vi "cube Controller.vi"(8 "error in":errorcluster) -> ()   [LabVIEW 2017]
doc: "This VI executes continuously carrying out the current operation and responding to updates or new operations. It will often contain the timing or control code that is difficult to place directly in TeleOp. This VI generally opens all sensors and motors and isolates the rest of the robot code from knowing how the operations are carried out."
uses:
  <vilib>/Rock Robotics/WPI/Framework/Completion Status.ctl
  cube Setpoints.ctl
  cube Operations.ctl
  <vilib>/Rock Robotics/WPI/MotorControl/WPI_MotorControlDeviceRef.ctl
  <vilib>/Rock Robotics/WPI/MotorControl/WPI_MotorControlType.ctl
  <vilib>/Rock Robotics/SystemInterfaces/DIO/FPGA_DIOPWMChannel.ctl
  <vilib>/Rock Robotics/WPI/PWM/WPI_PWMDeadband.ctl
  <vilib>/Rock Robotics/SystemInterfaces/DIO/FPGA_DIOChannel.ctl
  <vilib>/Rock Robotics/SystemInterfaces/AnalogTrigger/FPGA_AnalogTriggerDevRef.ctl
  <vilib>/Rock Robotics/SystemInterfaces/AnalogTrigger/FPGA_AnalogTriggerIndex.ctl
  cube Published Globals.vi
  <vilib>/Rock Robotics/SystemInterfaces/AI/FPGA_AIChannel.ctl
  Phoenix-LabVIEW/Motor Controller/Controls/CTRE_Phoenix_MotorControl_ControlMode.ctl
  Framework/Robot Global Data.vi
  <vilib>/Rock Robotics/Network Tables/NT Write Boolean.vi
panel:
  out "CubeLastCommandStatus":T1=enum."Incomplete"
  out "WaitTrigger":bool
  in  "Interactive Values":T2
  out "Current\nCmd":string
  in  "Buttons":cluster{"Execute Cmd":bool, "Abort Cmd":bool}
  out "Command Timing":cluster{"Start Time (ms)":u32, "Iterations":i32}
  out "Status":T1
  # "Tip: It may be helpful to observe inputs and sensor values.\nYou may also want to display tuning or debugging controls."
  # "Interactive Command: You may fill in the settings for a command\nand schedule it with the Execute button. You can observe and abort\nany command while fine tuning the code for the controller."
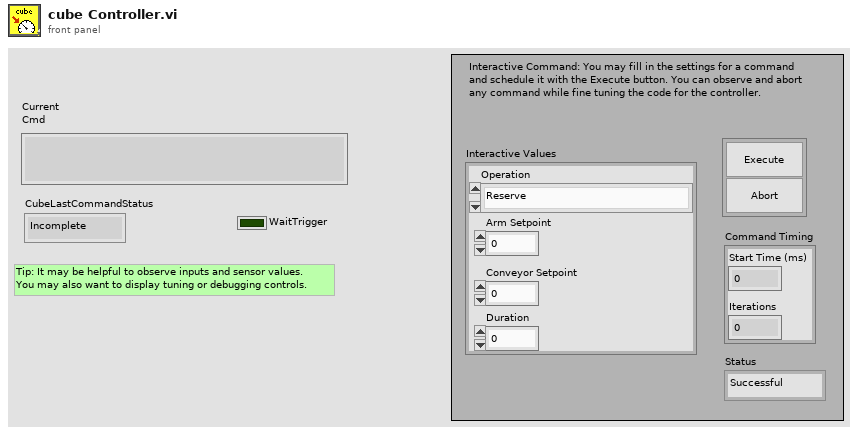
[diagram p1: front panel]
types:
  T1 = typedef "Completion Status.ctl" = enum16{"Successful", "Aborted", "Incomplete"}
  T2 = typedef "cube Setpoints.ctl" = cluster{"Operation":T3, "Arm Setpoint":dbl, "Duration":dbl, "Conveyor Setpoint":dbl}
  T3 = typedef "cube Operations.ctl" = enum16{"Reserve", "Read Current", "Immediate", "Chew", "Puke", "Swallow", "Poop", "SpitFast", "SpitSlow"}
  T4 = typedef "FPGA_AIChannel.ctl" = enum8{"AI 0", "AI 1", "AI 2", "AI 3", "AI MXP 0", "AI MXP 1", "AI MXP 2", "AI MXP 3", "Invalid"}
  T5 = typedef "FPGA_AnalogTriggerDevRef.ctl" = cluster{"DevStatus":errorcluster, "AnalogTriggerIndex":T6}
  T6 = typedef "FPGA_AnalogTriggerIndex.ctl" = enum8{"Trig 0", "Trig 1", "Trig 2", "Trig 3", "Trig 4", "Trig 5", "Trig 6", "Trig 7", "Invalid"}
  T7 = typedef "WPI_AnalogChannelDevRef.ctl" = cluster{"DevStatus":errorcluster, "Analog Channel":T4}
  T8 = typedef "WPI_MotorControlDeviceRef.ctl" = cluster{"DeviceStatus":errorcluster, "Type":T9, "PWM":cluster{"PWM Channel":T10, "DeadBand":T11}, "CAN":cluster{"Device Number":u8, "SetOutput VI Ref":variant, "GetOutput VI Ref":variant, "Enable VI Ref":variant, "Disable VI Ref":variant, "Data":variant}, "Invert":bool, "DIO PWM":cluster{"PWM \"Enable\" Channel":T10, "DIOChannel":T12, "PWM Rate":dbl}}
  T9 = typedef "WPI_MotorControlType.ctl" = enum16{"PWM", "CAN", "DIO PWM"}
  T10 = typedef "FPGA_DIOPWMChannel.ctl" = enum8{"PWM 0", "PWM 1", "PWM 2", "PWM 3", "PWM 4", "PWM 5", "PWM 6", "PWM 7", "PWM 8", "PWM 9", "PWM MXP 0", "PWM MXP 1", "PWM MXP 2", "PWM MXP 3", "PWM MXP 4", "PWM MXP 5", "PWM MXP 6", "PWM MXP 7", "PWM MXP 8", "PWM MXP 9", "Invalid"}
  T11 = typedef "WPI_PWMDeadband.ctl" = cluster{"Name":string, "maxPositivePwm":i32, "minPositivePwm":i32, "centerPwm":i32, "maxNegativePwm":i32, "minNegativePwm":i32, "angularRange":u16}
  T12 = typedef "FPGA_DIOChannel.ctl" = enum8{"DIO 0", "DIO 1", "DIO 2", "DIO 3", "DIO 4", "DIO 5", "DIO 6", "DIO 7", "DIO 8", "DIO 9", "DIO MXP 0", "DIO MXP 1", "DIO MXP 2", "DIO MXP 3", "DIO MXP 4", "DIO MXP 5", "DIO MXP 6", "DIO MXP 7", "DIO MXP 8", "DIO MXP 9", "DIO MXP 10", "DIO MXP 11", "DIO MXP 12", "DIO MXP 13", "DIO MXP 14", "DIO MXP 15", "SPI Port CS1", "SPI Port CS2", "SPI Port CS3", "SPI Port MISO", "SPI Port MOSI", "Invalid"}
  T13 = typedef "Command Status Info.ctl" = cluster{"Name":string, "Status":T1, "notifier out":T14}
  T14 = typedef "Completion Notifier.ctl" = refnum<notifier>
  T15 = cluster{"Current Command":T2, "Command Timing":cluster{"Start Time (ms)":u32, "Iterations":i32}, "Command Arguments":cluster{"Command Info":T13, "Description":string, "Default Command":T2, "queue out":refnum<queue>, "Subsystem Name":string}}
  T16 = typedef "CTRE_Phoenix_MotorControl_ControlMode.ctl" = u16
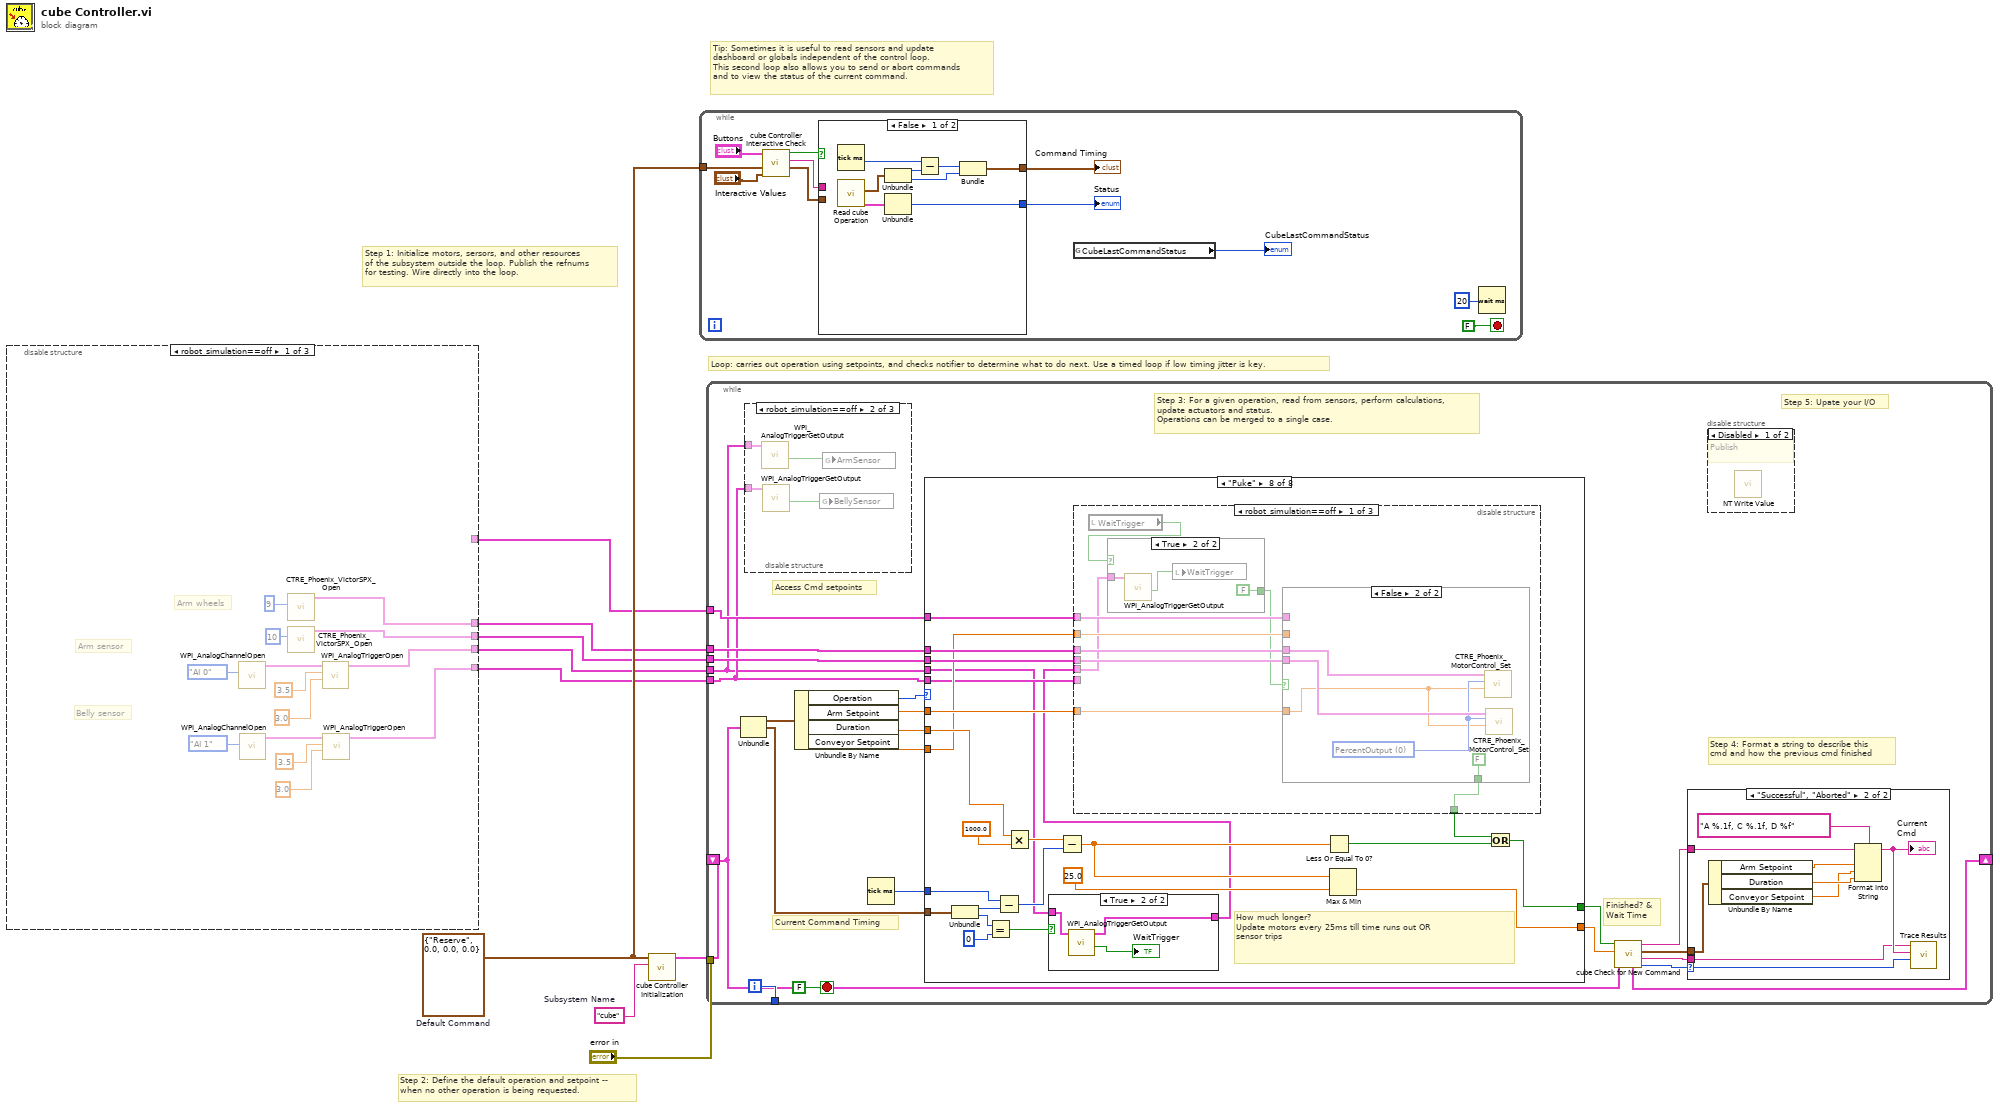
[diagram p0: block diagram]
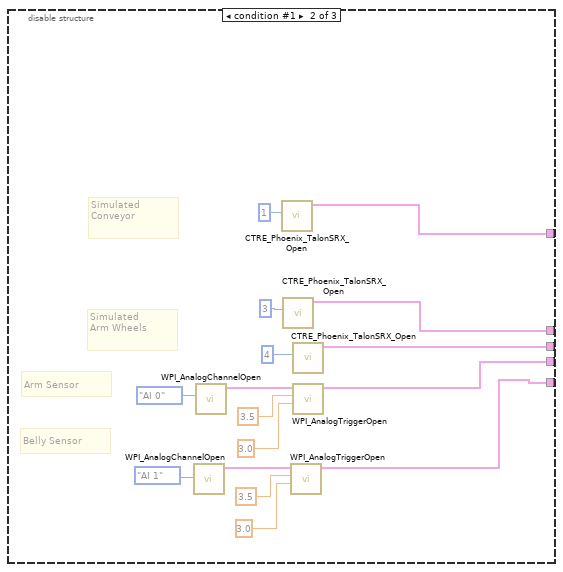
[diagram p2: hidden frame]
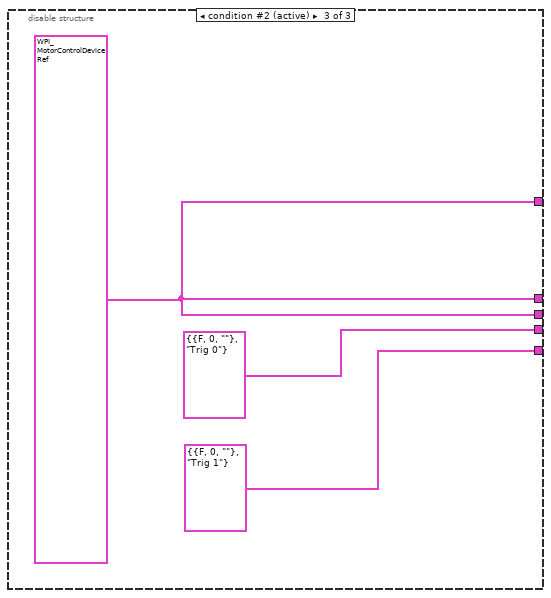
[diagram p3: hidden frame]
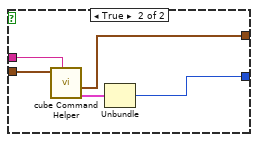
[diagram p4: hidden frame]
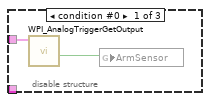
[diagram p5: hidden frame]
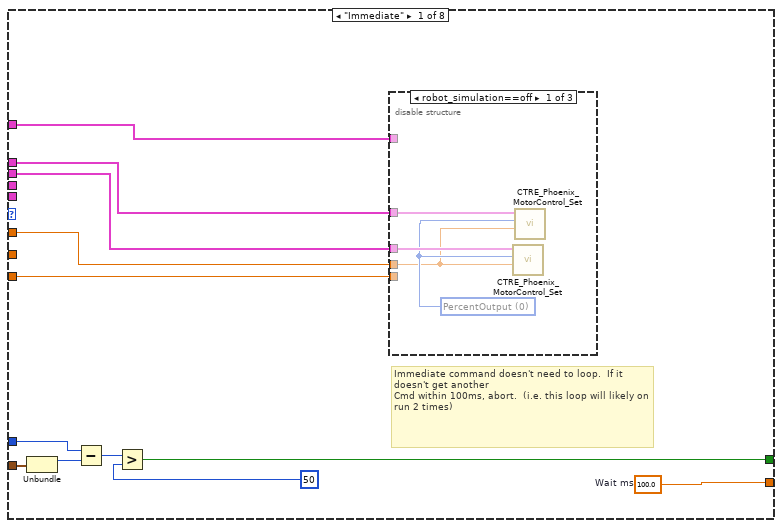
[diagram p9: hidden frame]
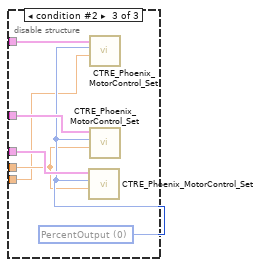
[diagram p11: hidden frame]
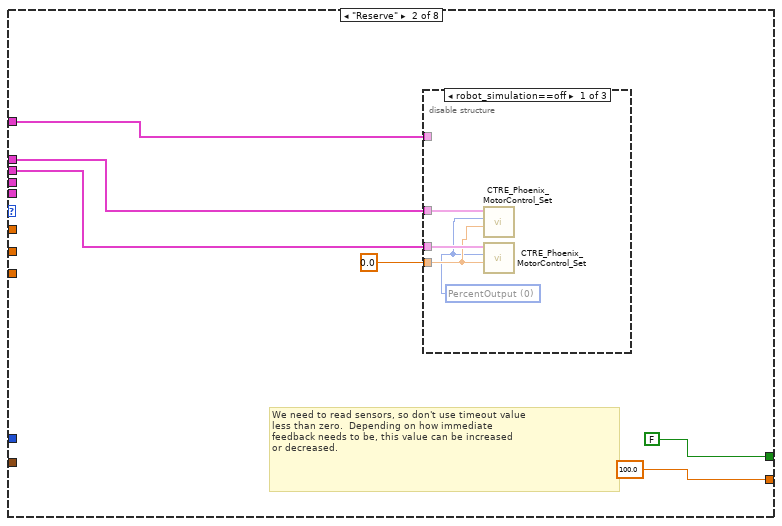
[diagram p12: hidden frame]
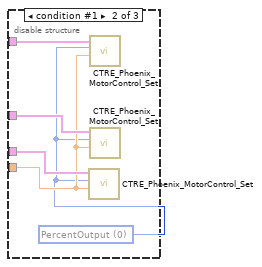
[diagram p13: hidden frame]
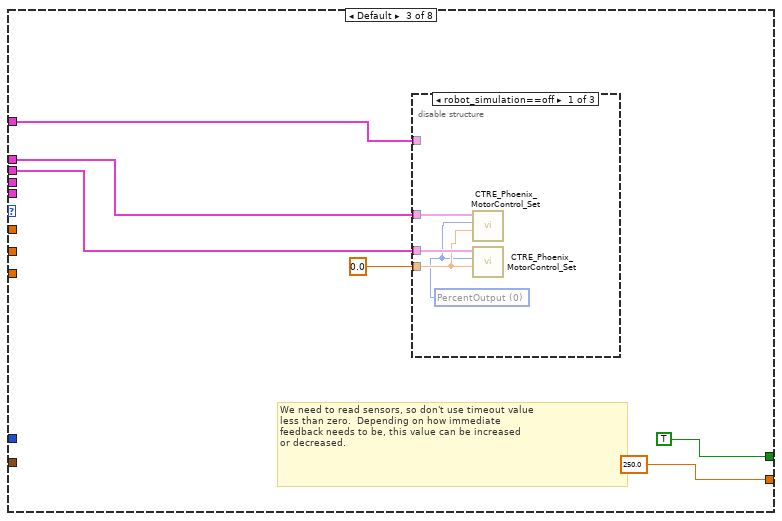
[diagram p15: hidden frame]
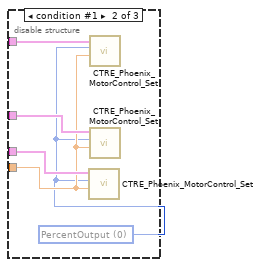
[diagram p16: hidden frame]
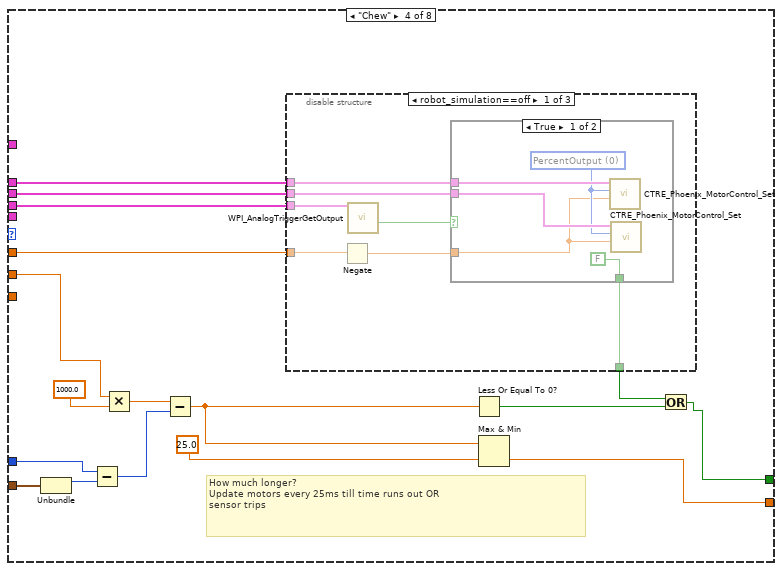
[diagram p18: hidden frame]
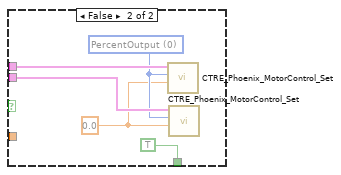
[diagram p19: hidden frame]
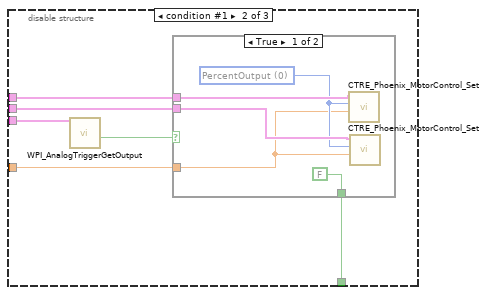
[diagram p20: hidden frame]
diagram:
  w6 = T2 {"Operation"=enum."Reserve", "Arm Setpoint"=0.0, "Duration"=0.0, "Conveyor Setpoint"=0.0}  # Default Command
  w7 = "cube"  # Subsystem Name
  # "Tip: Sometimes it is useful to read sensors and update\ndashboard or globals independent of the control loop.\nThis second loop also allows you to send or abort commands\nand to view the status of the current command."
  # "Step 2: Define the default operation and setpoint --\nwhen no other operation is being requested."
  # "Step 1: Initialize motors, sersors, and other resources\nof the subsystem outside the loop. Publish the refnums\nfor testing. Wire directly into the loop."
  # "Loop: carries out operation using setpoints, and checks notifier to determine what to do next. Use a timed loop if low timing jitter is key."
  n1 = disable-structure shown="robot_simulation==off" {
    disable-tunnel: [w21 w36 w42] -> w5
    disable-tunnel: [w20 w35 w42] -> w4
    disable-tunnel: [_ w34 w42] -> w1
    disable-tunnel: [w15 w29 T5 {"DevStatus"={"status"=FALSE, "code"=0, "source"=""}, "AnalogTriggerIndex"=enum."Trig 0"} ("AnalogTriggerDevRef")] -> w3
    disable-tunnel: [w10 w24 T5 {"DevStatus"={"status"=FALSE, "code"=0, "source"=""}, "AnalogTriggerIndex"=enum."Trig 1"} ("AnalogTriggerDevRef")] -> w2
    frame condition #0 {
      # "Belly sensor"
      # "Arm sensor"
      # "Arm wheels"
      n2 = call <vilib>:"WPI_AnalogChannelOpen.vi"("Analog Channel"=FPGA_AIChannel."AI 0") -> ("AIDeviceRef"=w18:T7)  [unwired: 9 in, 1 out]
      n3 = call <vilib>:"WPI_AnalogChannelOpen.vi"("Analog Channel"=FPGA_AIChannel."AI 1") -> ("AIDeviceRef"=w13:T7)  [unwired: 9 in, 1 out]
      n4 = call "CTRE_Phoenix_VictorSPX_Open.vi"("Device Number"=u8 9) -> ("CAN Talon SRX Ref"=w21:T8)  [unwired: 9 in, 1 out]
      n5 = call "CTRE_Phoenix_VictorSPX_Open.vi"("Device Number"=u8 10) -> ("CAN Talon SRX Ref"=w20:T8)  [unwired: 9 in, 1 out]
      n6 = call <vilib>:"WPI_AnalogTriggerOpen.vi"("LowerLimit (v)"=3.0, "UpperLimit (v)"=3.5, "AnalogTriggerSource"=w18) -> ("AnalogTriggerDevRef"=w15:T5)  [unwired: 7 in, 1 out]
      n7 = call <vilib>:"WPI_AnalogTriggerOpen.vi"("LowerLimit (v)"=3.0, "UpperLimit (v)"=3.5, "AnalogTriggerSource"=w13) -> ("AnalogTriggerDevRef"=w10:T5)  [unwired: 7 in, 1 out]
    }
    frame condition #1 {
      # "Belly Sensor"
      # "Arm Sensor"
      # "Simulated\nConveyor"
      # "Simulated\nArm Wheels"
      n8 = call <vilib>:"WPI_AnalogChannelOpen.vi"("Analog Channel"=FPGA_AIChannel."AI 1") -> ("AIDeviceRef"=w27:T7)  [unwired: 9 in, 1 out]
      n9 = call <vilib>:"WPI_AnalogChannelOpen.vi"("Analog Channel"=FPGA_AIChannel."AI 0") -> ("AIDeviceRef"=w32:T7)  [unwired: 9 in, 1 out]
      n10 = call "CTRE_Phoenix_TalonSRX_Open.vi"("Device Number"=u8 1) -> ("CAN Talon SRX Ref"=w34:T8)  [unwired: 9 in, 1 out]
      n11 = call "CTRE_Phoenix_TalonSRX_Open.vi"("Device Number"=u8 3) -> ("CAN Talon SRX Ref"=w36:T8)  [unwired: 9 in, 1 out]
      n12 = call <vilib>:"WPI_AnalogTriggerOpen.vi"("LowerLimit (v)"=3.0, "UpperLimit (v)"=3.5, "AnalogTriggerSource"=w27) -> ("AnalogTriggerDevRef"=w24:T5)  [unwired: 7 in, 1 out]
      n13 = call "CTRE_Phoenix_TalonSRX_Open.vi"("Device Number"=u8 4) -> ("CAN Talon SRX Ref"=w35:T8)  [unwired: 9 in, 1 out]
      n14 = call <vilib>:"WPI_AnalogTriggerOpen.vi"("LowerLimit (v)"=3.0, "UpperLimit (v)"=3.5, "AnalogTriggerSource"=w32) -> ("AnalogTriggerDevRef"=w29:T5)  [unwired: 7 in, 1 out]
    }
    frame condition #2 (active) {
      w42 = T8 {"DeviceStatus"={"status"=FALSE, "code"=0, "source"=""}, "Type"=enum."PWM", "PWM"={"PWM Channel"=enum."Invalid", "DeadBand"={"Name"="", "maxPositivePwm"=0, "minPositivePwm"=0, "centerPwm"=0, "maxNegativePwm"=0, "minNegativePwm"=0, "angularRange"=0}}, "CAN"={"Device Number"=0, "SetOutput VI Ref"=variant, "GetOutput VI Ref"=variant, "Enable VI Ref"=variant, "Disable VI Ref"=variant, "Data"=variant}, "Invert"=FALSE, "DIO PWM"={"PWM \"Enable\" Channel"=enum."Invalid", "DIOChannel"=enum."Invalid", "PWM Rate"=0.0}} ("CAN Talon SRX Ref")
    }
  }
  n15 = call "cube Controller Initialization.vi"("Subsystem Name"=w7, "Default Command"=w6) -> ("Current Command"=w8:T15)  [unwired: 9 in]
  n16 = while {
    tunnel: w6 -> [w50]
    stop <- FALSE stop-if-true
    n17 = call "cube Controller Interactive Check.vi"("Interactive Command in"="Interactive Values", "Default Command"=w50, "Buttons"="Buttons") -> ("Interactive Command out"=w47:T2, "Trace String"=w48:string, "Schedule"=w49:bool)  [unwired: 6 in]
    n18 = case shown="False" w49 {
      tunnel: [w61 w66] -> w46
      tunnel: w47 -> [_ w64]
      tunnel: [w57 w62] -> w45
      tunnel: w48 -> [_ w65]
      frame False {
        n19 = Tick Count (ms)() -> (millisecond timer value=w56:u32)
        n20 = call "Read cube Operation.vi"() -> ("Command Info"=w55:T13, "Command Timing"=w54:cluster{"Start Time (ms)":u32, "Iterations":i32})  [unwired: 9 in, 1 out]
        n21 = Unbundle(w54) -> ("Start Time (ms)"=w60:u32, "Iterations"=w58:i32)
        n22 = Unbundle(w55) -> ("Status"=w61:T1)  [unwired: 2 out]
        n23 = Subtract(x=w56, y=w60) -> (x-y=w59:u32)
        n24 = Bundle(w59, "Iterations"=w58) -> (w57:cluster{u32, "Iterations":i32})  [unwired: 1 in]
      }
      frame True {
        n25 = call "cube Command Helper.vi"("Description"=w65, "SubSystem Data"=w64) -> ("Command Info Out"=w63:T13, "Command Timing"=w62:cluster{"Start Time (ms)":u32, "Iterations":i32})  [unwired: 7 in, 1 out]
        n26 = Unbundle(w63) -> ("Status"=w66:T1)  [unwired: 2 out]
      }
    }
    "Status" <- w46
    "Command Timing" <- w45
    n27 = global read "cube Published Globals.vi" "CubeLastCommandStatus"() -> (→"CubeLastCommandStatus":T1)
    n28 = Wait (ms)(milliseconds to wait=u32 20) -> ()  [unwired: 1 out]
  }
  n29 = while {
    shift-right: [w84] -> _
    shift-left: w8 -> [w79]
    tunnel: [w87] -> _
    tunnel: "error in" -> [_]
    tunnel: w5 -> [w78]
    tunnel: w4 -> [w77]
    tunnel: w1 -> [w76]
    tunnel: w3 -> [w69]
    tunnel: w2 -> [w70]
    i -> [w87]
    stop <- FALSE stop-if-true
    # "Step 5: Upate your I/O"
    # "Step 4: Format a string to describe this\ncmd and how the previous cmd finished"
    # "Current Command Timing"
    # "Access Cmd setpoints"
    # "Finished? &\nWait Time"
    # "Step 3: For a given operation, read from sensors, perform calculations,\nupdate actuators and status.\nOperations can be merged to a single case."
    n30 = Unbundle(w79) -> ("Current Command"=w75:T2, "Command Timing"=w85:cluster{"Start Time (ms)":u32, "Iterations":i32})  [unwired: 1 out]
    n31 = disable-structure shown="robot_simulation==off" {
      disable-tunnel: w70 -> [_ w92 _]
      disable-tunnel: w69 -> [w89 w91 _]
      frame condition #0 {
        n32 = call <vilib>:"WPI_AnalogTriggerGetOutput.vi"("AnalogTriggerDevRef"=w89) -> ("Trigger State"=w90:bool)  [unwired: 7 in, 3 out]
        n33 = global write "Robot Global Data.vi" "ArmSensor"(w90) -> ()
      }
      frame condition #1 {
        n34 = call <vilib>:"WPI_AnalogTriggerGetOutput.vi"("AnalogTriggerDevRef"=w91) -> ("Trigger State"=w94:bool)  [unwired: 7 in, 3 out]
        n35 = call <vilib>:"WPI_AnalogTriggerGetOutput.vi"("AnalogTriggerDevRef"=w92) -> ("Trigger State"=w93:bool)  [unwired: 7 in, 3 out]
        n36 = global write "Robot Global Data.vi" "BellySensor"(w93) -> ()
        n37 = global write "Robot Global Data.vi" "ArmSensor"(w94) -> ()
      }
      frame condition #2 (active) {
      }
    }
    n38 = Unbundle By Name(w75) -> ("Operation"=w74:T3, "Arm Setpoint"=w73:dbl, "Duration"=w72:dbl, "Conveyor Setpoint"=w71:dbl)
    n39 = Tick Count (ms)() -> (millisecond timer value=w86:u32)
    n40 = case shown="\"Puke\"" w74 {
      tunnel: [w115 100.0 250.0 ("Infinite") w164 w216 w248 w278 w343] -> w67
      tunnel: [w109 FALSE ("ignore previous (F)") TRUE ("ignore previous (F)") w159 w212 w243 w274 w339] -> w68
      tunnel: w85 -> [w111 _ _ w166 w218 w250 w280 w345]
      tunnel: w86 -> [w110 _ _ w165 w217 w249 w279 w344]
      tunnel: w78 -> [w107 w128 w143 w163 w215 w247 w277 w342]
      tunnel: w77 -> [w106 w127 w142 w162 w214 w246 w276 w341]
      tunnel: w76 -> [w108 w129 w144 _ w207 _ w269 w335]
      tunnel: w73 -> [w105 _ _ w156 w209 w240 w271 w336]
      tunnel: w72 -> [_ _ _ w161 w213 w245 w275 w340]
      tunnel: w71 -> [w104 _ _ _ w206 _ w268 w334]
      tunnel: w69 -> [_ _ _ w160 _ w244 _ w329]
      tunnel: w70 -> [_ _ _ _ w208 _ w270 w333]
      frame "Immediate" {
        w115 = 100.0  # Wait ms
        # "Immediate command doesn't need to loop.  If it doesn't get another\nCmd within 100ms, abort.  (i.e. this loop will likely on run 2 times)"
        n41 = Unbundle(w111) -> ("Start Time (ms)"=w114:u32)  [unwired: 1 out]
        n42 = Subtract(x=w110, y=w114) -> (x-y=w113:u32)
        n43 = Greater?(x=w113, y=u8 50 ("Left Motor")) -> (0:w109:bool)
        n44 = disable-structure shown="robot_simulation==off" {
          disable-tunnel: w108 -> [_ _ w125]
          disable-tunnel: w107 -> [w119 _ w124]
          disable-tunnel: w106 -> [w118 _ w123]
          disable-tunnel: w105 -> [w116 _ w121]
          disable-tunnel: w104 -> [_ _ w120]
          frame condition #0 {
            w117 = T16 0 items=["PercentOutput"=0, "Position"=1, "Velocity"=2, "Current"=3, "Follower"=5, "MotionProfile"=6, "MotionMagic"=7, "MotionMagicArc"=8, "MotionProfileArc"=10, "Disabled"=15] ("Control Mode")
            n45 = call "CTRE_Phoenix_MotorControl_Set.vi"("Output"=w116, "Control Mode"=w117, "PhoenixMotorControlDevRef"=w118) -> ()  [unwired: 7 in, 2 out]
            n46 = call "CTRE_Phoenix_MotorControl_Set.vi"("Output"=w116, "Control Mode"=w117, "PhoenixMotorControlDevRef"=w119) -> ()  [unwired: 7 in, 2 out]
          }
          frame condition #1 (active) {
          }
          frame condition #2 {
            w122 = T16 0 items=["PercentOutput"=0, "Position"=1, "Velocity"=2, "Current"=3, "Follower"=5, "MotionProfile"=6, "MotionMagic"=7, "MotionMagicArc"=8, "MotionProfileArc"=10, "Disabled"=15] ("Control Mode")
            n47 = call "CTRE_Phoenix_MotorControl_Set.vi"("Output"=w121, "Control Mode"=w122, "PhoenixMotorControlDevRef"=w123) -> ()  [unwired: 7 in, 2 out]
            n48 = call "CTRE_Phoenix_MotorControl_Set.vi"("Output"=w120, "Control Mode"=w122, "PhoenixMotorControlDevRef"=w125) -> ()  [unwired: 7 in, 2 out]
            n49 = call "CTRE_Phoenix_MotorControl_Set.vi"("Output"=w121, "Control Mode"=w122, "PhoenixMotorControlDevRef"=w124) -> ()  [unwired: 7 in, 2 out]
          }
        }
      }
      frame "Reserve" {
        # "We need to read sensors, so don't use timeout value\nless than zero.  Depending on how immediate \nfeedback needs to be, this value can be increased\nor decreased."
        n50 = disable-structure shown="robot_simulation==off" {
          disable-tunnel: w129 -> [_ w140 _]
          disable-tunnel: w128 -> [w135 w139 _]
          disable-tunnel: w127 -> [w134 w138 _]
          disable-tunnel: 0.0 ("Setpoint") -> [w133 w137 _]
          frame condition #0 {
            w132 = T16 0 items=["PercentOutput"=0, "Position"=1, "Velocity"=2, "Current"=3, "Follower"=5, "MotionProfile"=6, "MotionMagic"=7, "MotionMagicArc"=8, "MotionProfileArc"=10, "Disabled"=15] ("Control Mode")
            n51 = call "CTRE_Phoenix_MotorControl_Set.vi"("Output"=w133, "Control Mode"=w132, "PhoenixMotorControlDevRef"=w135) -> ()  [unwired: 7 in, 2 out]
            n52 = call "CTRE_Phoenix_MotorControl_Set.vi"("Output"=w133, "Control Mode"=w132, "PhoenixMotorControlDevRef"=w134) -> ()  [unwired: 7 in, 2 out]
          }
          frame condition #1 {
            w136 = T16 0 items=["PercentOutput"=0, "Position"=1, "Velocity"=2, "Current"=3, "Follower"=5, "MotionProfile"=6, "MotionMagic"=7, "MotionMagicArc"=8, "MotionProfileArc"=10, "Disabled"=15] ("Control Mode")
            n53 = call "CTRE_Phoenix_MotorControl_Set.vi"("Output"=w137, "Control Mode"=w136, "PhoenixMotorControlDevRef"=w138) -> ()  [unwired: 7 in, 2 out]
            n54 = call "CTRE_Phoenix_MotorControl_Set.vi"("Output"=w137, "Control Mode"=w136, "PhoenixMotorControlDevRef"=w140) -> ()  [unwired: 7 in, 2 out]
            n55 = call "CTRE_Phoenix_MotorControl_Set.vi"("Output"=w137, "Control Mode"=w136, "PhoenixMotorControlDevRef"=w139) -> ()  [unwired: 7 in, 2 out]
          }
          frame condition #2 (active) {
          }
        }
      }
      frame Default {
        # "We need to read sensors, so don't use timeout value\nless than zero.  Depending on how immediate \nfeedback needs to be, this value can be increased\nor decreased."
        n56 = disable-structure shown="robot_simulation==off" {
          disable-tunnel: w144 -> [_ w155 _]
          disable-tunnel: w143 -> [w150 w154 _]
          disable-tunnel: w142 -> [w149 w153 _]
          disable-tunnel: 0.0 ("Setpoint") -> [w148 w152 _]
          frame condition #0 {
            w147 = T16 0 items=["PercentOutput"=0, "Position"=1, "Velocity"=2, "Current"=3, "Follower"=5, "MotionProfile"=6, "MotionMagic"=7, "MotionMagicArc"=8, "MotionProfileArc"=10, "Disabled"=15] ("Control Mode")
            n57 = call "CTRE_Phoenix_MotorControl_Set.vi"("Output"=w148, "Control Mode"=w147, "PhoenixMotorControlDevRef"=w150) -> ()  [unwired: 7 in, 2 out]
            n58 = call "CTRE_Phoenix_MotorControl_Set.vi"("Output"=w148, "Control Mode"=w147, "PhoenixMotorControlDevRef"=w149) -> ()  [unwired: 7 in, 2 out]
          }
          frame condition #1 {
            w151 = T16 0 items=["PercentOutput"=0, "Position"=1, "Velocity"=2, "Current"=3, "Follower"=5, "MotionProfile"=6, "MotionMagic"=7, "MotionMagicArc"=8, "MotionProfileArc"=10, "Disabled"=15] ("Control Mode")
            n59 = call "CTRE_Phoenix_MotorControl_Set.vi"("Output"=w152, "Control Mode"=w151, "PhoenixMotorControlDevRef"=w153) -> ()  [unwired: 7 in, 2 out]
            n60 = call "CTRE_Phoenix_MotorControl_Set.vi"("Output"=w152, "Control Mode"=w151, "PhoenixMotorControlDevRef"=w155) -> ()  [unwired: 7 in, 2 out]
            n61 = call "CTRE_Phoenix_MotorControl_Set.vi"("Output"=w152, "Control Mode"=w151, "PhoenixMotorControlDevRef"=w154) -> ()  [unwired: 7 in, 2 out]
          }
          frame condition #2 (active) {
          }
        }
      }
      frame "Chew" {
        # "How much longer?\nUpdate motors every 25ms till time runs out OR\nsensor trips"
        n62 = Unbundle(w166) -> ("Start Time (ms)"=w169:u32)  [unwired: 1 out]
        n63 = Subtract(x=w165, y=w169) -> (x-y=w172:u32)
        n64 = Multiply(x=w161, y=1000.0) -> (x*y=w171:dbl)
        n65 = Subtract(x=w171, y=w172) -> (x-y=w168:dbl)
        n66 = disable-structure shown="robot_simulation==off" {
          disable-tunnel: w163 -> [w179 w195 _]
          disable-tunnel: w162 -> [w178 w194 _]
          disable-tunnel: w156 -> [w173 w193 _]
          disable-tunnel: w160 -> [w177 w192 _]
          disable-tunnel: [w175 w190 _] -> w157
          frame condition #0 {
            n67 = Negate(x=w173) -> (-x=w174:dbl)
            n68 = call <vilib>:"WPI_AnalogTriggerGetOutput.vi"("AnalogTriggerDevRef"=w177) -> ("Trigger State"=w176:bool)  [unwired: 7 in, 3 out]
            n69 = case shown="True" w176 {
              tunnel: w179 -> [w184 w189]
              tunnel: w178 -> [w183 w188]
              tunnel: w174 -> [w180 _]
              tunnel: [FALSE TRUE] -> w175
              frame True {
                w182 = T16 0 items=["PercentOutput"=0, "Position"=1, "Velocity"=2, "Current"=3, "Follower"=5, "MotionProfile"=6, "MotionMagic"=7, "MotionMagicArc"=8, "MotionProfileArc"=10, "Disabled"=15] ("Control Mode")
                n70 = call "CTRE_Phoenix_MotorControl_Set.vi"("Output"=w180, "Control Mode"=w182, "PhoenixMotorControlDevRef"=w184) -> ()  [unwired: 7 in, 2 out]
                n71 = call "CTRE_Phoenix_MotorControl_Set.vi"("Output"=w180, "Control Mode"=w182, "PhoenixMotorControlDevRef"=w183) -> ()  [unwired: 7 in, 2 out]
              }
              frame False {
                w186 = 0.0 ("Output")
                w187 = T16 0 items=["PercentOutput"=0, "Position"=1, "Velocity"=2, "Current"=3, "Follower"=5, "MotionProfile"=6, "MotionMagic"=7, "MotionMagicArc"=8, "MotionProfileArc"=10, "Disabled"=15] ("Control Mode")
                n72 = call "CTRE_Phoenix_MotorControl_Set.vi"("Output"=w186, "Control Mode"=w187, "PhoenixMotorControlDevRef"=w189) -> ()  [unwired: 7 in, 2 out]
                n73 = call "CTRE_Phoenix_MotorControl_Set.vi"("Output"=w186, "Control Mode"=w187, "PhoenixMotorControlDevRef"=w188) -> ()  [unwired: 7 in, 2 out]
              }
            }
          }
          frame condition #1 {
            n74 = call <vilib>:"WPI_AnalogTriggerGetOutput.vi"("AnalogTriggerDevRef"=w192) -> ("Trigger State"=w191:bool)  [unwired: 7 in, 3 out]
            n75 = case shown="True" w191 {
              tunnel: w195 -> [w199 w205]
              tunnel: w194 -> [w198 w204]
              tunnel: w193 -> [w196 _]
              tunnel: [FALSE TRUE] -> w190
              frame True {
                w197 = T16 0 items=["PercentOutput"=0, "Position"=1, "Velocity"=2, "Current"=3, "Follower"=5, "MotionProfile"=6, "MotionMagic"=7, "MotionMagicArc"=8, "MotionProfileArc"=10, "Disabled"=15] ("Control Mode")
                n76 = call "CTRE_Phoenix_MotorControl_Set.vi"("Output"=w196, "Control Mode"=w197, "PhoenixMotorControlDevRef"=w199) -> ()  [unwired: 7 in, 2 out]
                n77 = call "CTRE_Phoenix_MotorControl_Set.vi"("Output"=w196, "Control Mode"=w197, "PhoenixMotorControlDevRef"=w198) -> ()  [unwired: 7 in, 2 out]
              }
              frame False {
                w203 = T16 0 items=["PercentOutput"=0, "Position"=1, "Velocity"=2, "Current"=3, "Follower"=5, "MotionProfile"=6, "MotionMagic"=7, "MotionMagicArc"=8, "MotionProfileArc"=10, "Disabled"=15] ("Control Mode")
                w202 = 0.0 ("Output")
                n78 = call "CTRE_Phoenix_MotorControl_Set.vi"("Output"=w202, "Control Mode"=w203, "PhoenixMotorControlDevRef"=w205) -> ()  [unwired: 7 in, 2 out]
                n79 = call "CTRE_Phoenix_MotorControl_Set.vi"("Output"=w202, "Control Mode"=w203, "PhoenixMotorControlDevRef"=w204) -> ()  [unwired: 7 in, 2 out]
              }
            }
          }
          frame condition #2 (active) {
          }
        }
        n80 = Less Or Equal To 0?(x=w168) -> (x <= 0?=w158:bool)
        n81 = Max & Min(x=w168, y=25.0) -> (min(x,y)=w164:dbl)  [unwired: 1 out]
        n82 = Or(x=w157, y=w158) -> (x .or. y?=w159:bool)
      }
      frame "Poop" {
        # "How much longer?\nUpdate motors every 25ms till time runs out OR\nsensor trips"
        n83 = Unbundle(w218) -> ("Start Time (ms)"=w221:u32)  [unwired: 1 out]
        n84 = Subtract(x=w217, y=w221) -> (x-y=w224:u32)
        n85 = Multiply(x=w213, y=1000.0) -> (x*y=w223:dbl)
        n86 = Subtract(x=w223, y=w224) -> (x-y=w220:dbl)
        n87 = disable-structure shown="robot_simulation==off" {
          disable-tunnel: w215 -> [w230 w239 _]
          disable-tunnel: w214 -> [w229 w238 _]
          disable-tunnel: w209 -> [w227 w234 _]
          disable-tunnel: w208 -> [_ _ _]
          disable-tunnel: [FALSE FALSE _] -> w210
          disable-tunnel: w207 -> [_ w236 _]
          disable-tunnel: w206 -> [_ w233 _]
          frame condition #0 {
            w226 = T16 0 items=["PercentOutput"=0, "Position"=1, "Velocity"=2, "Current"=3, "Follower"=5, "MotionProfile"=6, "MotionMagic"=7, "MotionMagicArc"=8, "MotionProfileArc"=10, "Disabled"=15] ("Control Mode")
            n88 = Negate(x=w227) -> (-x=w225:dbl)
            n89 = call "CTRE_Phoenix_MotorControl_Set.vi"("Output"=w225, "Control Mode"=w226, "PhoenixMotorControlDevRef"=w230) -> ()  [unwired: 7 in, 2 out]
            n90 = call "CTRE_Phoenix_MotorControl_Set.vi"("Output"=w225, "Control Mode"=w226, "PhoenixMotorControlDevRef"=w229) -> ()  [unwired: 7 in, 2 out]
          }
          frame condition #1 {
            w235 = T16 0 items=["PercentOutput"=0, "Position"=1, "Velocity"=2, "Current"=3, "Follower"=5, "MotionProfile"=6, "MotionMagic"=7, "MotionMagicArc"=8, "MotionProfileArc"=10, "Disabled"=15] ("Control Mode")
            n91 = Negate(x=w234) -> (-x=w231:dbl)
            n92 = Negate(x=w233) -> (-x=w232:dbl)
            n93 = call "CTRE_Phoenix_MotorControl_Set.vi"("Output"=w231, "Control Mode"=w235, "PhoenixMotorControlDevRef"=w239) -> ()  [unwired: 7 in, 2 out]
            n94 = call "CTRE_Phoenix_MotorControl_Set.vi"("Output"=w231, "Control Mode"=w235, "PhoenixMotorControlDevRef"=w238) -> ()  [unwired: 7 in, 2 out]
            n95 = call "CTRE_Phoenix_MotorControl_Set.vi"("Output"=w232, "Control Mode"=w235, "PhoenixMotorControlDevRef"=w236) -> ()  [unwired: 7 in, 2 out]
          }
          frame condition #2 (active) {
          }
        }
        n96 = Less Or Equal To 0?(x=w220) -> (x <= 0?=w211:bool)
        n97 = Max & Min(x=w220, y=25.0) -> (min(x,y)=w216:dbl)  [unwired: 1 out]
        n98 = Or(x=w210, y=w211) -> (x .or. y?=w212:bool)
      }
      frame "SpitFast" {
        # "How much longer?\nUpdate motors every 25ms till time runs out OR\nsensor trips"
        n99 = Unbundle(w250) -> ("Start Time (ms)"=w253:u32)  [unwired: 1 out]
        n100 = Subtract(x=w249, y=w253) -> (x-y=w256:u32)
        n101 = Multiply(x=w245, y=1000.0) -> (x*y=w255:dbl)
        n102 = Subtract(x=w255, y=w256) -> (x-y=w252:dbl)
        n103 = disable-structure shown="robot_simulation==off" {
          disable-tunnel: w247 -> [w261 w267 _]
          disable-tunnel: w246 -> [w260 w266 _]
          disable-tunnel: w240 -> [w257 w264 _]
          disable-tunnel: w244 -> [_ _ _]
          disable-tunnel: [FALSE FALSE _] -> w241
          frame condition #0 {
            w258 = T16 0 items=["PercentOutput"=0, "Position"=1, "Velocity"=2, "Current"=3, "Follower"=5, "MotionProfile"=6, "MotionMagic"=7, "MotionMagicArc"=8, "MotionProfileArc"=10, "Disabled"=15] ("Control Mode")
            n104 = call "CTRE_Phoenix_MotorControl_Set.vi"("Output"=w257, "Control Mode"=w258, "PhoenixMotorControlDevRef"=w261) -> ()  [unwired: 7 in, 2 out]
            n105 = call "CTRE_Phoenix_MotorControl_Set.vi"("Output"=w257, "Control Mode"=w258, "PhoenixMotorControlDevRef"=w260) -> ()  [unwired: 7 in, 2 out]
          }
          frame condition #1 {
            w263 = T16 0 items=["PercentOutput"=0, "Position"=1, "Velocity"=2, "Current"=3, "Follower"=5, "MotionProfile"=6, "MotionMagic"=7, "MotionMagicArc"=8, "MotionProfileArc"=10, "Disabled"=15] ("Control Mode")
            n106 = Negate(x=w264) -> (-x=w262:dbl)
            n107 = call "CTRE_Phoenix_MotorControl_Set.vi"("Output"=w262, "Control Mode"=w263, "PhoenixMotorControlDevRef"=w267) -> ()  [unwired: 7 in, 2 out]
            n108 = call "CTRE_Phoenix_MotorControl_Set.vi"("Output"=w262, "Control Mode"=w263, "PhoenixMotorControlDevRef"=w266) -> ()  [unwired: 7 in, 2 out]
          }
          frame condition #2 (active) {
          }
        }
        n109 = Less Or Equal To 0?(x=w252) -> (x <= 0?=w242:bool)
        n110 = Max & Min(x=w252, y=25.0) -> (min(x,y)=w248:dbl)  [unwired: 1 out]
        n111 = Or(x=w241, y=w242) -> (x .or. y?=w243:bool)
      }
      frame "Swallow" {
        # "How much longer?\nUpdate motors every 25ms till time runs out OR\nsensor trips"
        n112 = Unbundle(w280) -> ("Start Time (ms)"=w283:u32)  [unwired: 1 out]
        n113 = Subtract(x=w279, y=w283) -> (x-y=w286:u32)
        n114 = Multiply(x=w275, y=1000.0) -> (x*y=w285:dbl)
        n115 = Subtract(x=w285, y=w286) -> (x-y=w282:dbl)
        n116 = disable-structure shown="robot_simulation==off" {
          disable-tunnel: w277 -> [w293 w314 _]
          disable-tunnel: w276 -> [w292 w313 _]
          disable-tunnel: w271 -> [w288 w312 _]
          disable-tunnel: w270 -> [w295 w311 _]
          disable-tunnel: [w291 w309 _] -> w272
          disable-tunnel: w269 -> [w294 w308 _]
          disable-tunnel: w268 -> [w289 w307 _]
          frame condition #0 {
            n117 = Negate(x=w288) -> (-x=w287:dbl)
            n118 = call <vilib>:"WPI_AnalogTriggerGetOutput.vi"("AnalogTriggerDevRef"=w295) -> ("Trigger State"=w290:bool)  [unwired: 7 in, 3 out]
            n119 = case shown="True" w290 {
              tunnel: w293 -> [w299 w306]
              tunnel: w292 -> [w298 w305]
              tunnel: w287 -> [w296 _]
              tunnel: [FALSE TRUE] -> w291
              tunnel: w294 -> [_ w303]
              tunnel: w289 -> [_ _]
              frame True {
                w297 = T16 0 items=["PercentOutput"=0, "Position"=1, "Velocity"=2, "Current"=3, "Follower"=5, "MotionProfile"=6, "MotionMagic"=7, "MotionMagicArc"=8, "MotionProfileArc"=10, "Disabled"=15] ("Control Mode")
                n120 = call "CTRE_Phoenix_MotorControl_Set.vi"("Output"=w296, "Control Mode"=w297, "PhoenixMotorControlDevRef"=w299) -> ()  [unwired: 7 in, 2 out]
                n121 = call "CTRE_Phoenix_MotorControl_Set.vi"("Output"=w296, "Control Mode"=w297, "PhoenixMotorControlDevRef"=w298) -> ()  [unwired: 7 in, 2 out]
              }
              frame False {
                w301 = T16 0 items=["PercentOutput"=0, "Position"=1, "Velocity"=2, "Current"=3, "Follower"=5, "MotionProfile"=6, "MotionMagic"=7, "MotionMagicArc"=8, "MotionProfileArc"=10, "Disabled"=15] ("Control Mode")
                w302 = 0.0 ("Output")
                n122 = call "CTRE_Phoenix_MotorControl_Set.vi"("Output"=w302, "Control Mode"=w301, "PhoenixMotorControlDevRef"=w303) -> ()  [unwired: 7 in, 2 out]
                n123 = call "CTRE_Phoenix_MotorControl_Set.vi"("Output"=w302, "Control Mode"=w301, "PhoenixMotorControlDevRef"=w306) -> ()  [unwired: 7 in, 2 out]
                n124 = call "CTRE_Phoenix_MotorControl_Set.vi"("Output"=w302, "Control Mode"=w301, "PhoenixMotorControlDevRef"=w305) -> ()  [unwired: 7 in, 2 out]
              }
            }
          }
          frame condition #1 {
            n125 = call <vilib>:"WPI_AnalogTriggerGetOutput.vi"("AnalogTriggerDevRef"=w311) -> ("Trigger State"=w310:bool)  [unwired: 7 in, 3 out]
            n126 = case shown="True" w310 {
              tunnel: w314 -> [w320 w327]
              tunnel: w313 -> [w319 w326]
              tunnel: w312 -> [w315 _]
              tunnel: [FALSE TRUE] -> w309
              tunnel: w308 -> [w318 w324]
              tunnel: w307 -> [w316 _]
              frame True {
                w317 = T16 0 items=["PercentOutput"=0, "Position"=1, "Velocity"=2, "Current"=3, "Follower"=5, "MotionProfile"=6, "MotionMagic"=7, "MotionMagicArc"=8, "MotionProfileArc"=10, "Disabled"=15] ("Control Mode")
                n127 = call "CTRE_Phoenix_MotorControl_Set.vi"("Output"=w315, "Control Mode"=w317, "PhoenixMotorControlDevRef"=w320) -> ()  [unwired: 7 in, 2 out]
                n128 = call "CTRE_Phoenix_MotorControl_Set.vi"("Output"=w315, "Control Mode"=w317, "PhoenixMotorControlDevRef"=w319) -> ()  [unwired: 7 in, 2 out]
                n129 = call "CTRE_Phoenix_MotorControl_Set.vi"("Output"=w316, "Control Mode"=w317, "PhoenixMotorControlDevRef"=w318) -> ()  [unwired: 7 in, 2 out]
              }
              frame False {
                w322 = T16 0 items=["PercentOutput"=0, "Position"=1, "Velocity"=2, "Current"=3, "Follower"=5, "MotionProfile"=6, "MotionMagic"=7, "MotionMagicArc"=8, "MotionProfileArc"=10, "Disabled"=15] ("Control Mode")
                w323 = 0.0 ("Output")
                n130 = call "CTRE_Phoenix_MotorControl_Set.vi"("Output"=w323, "Control Mode"=w322, "PhoenixMotorControlDevRef"=w324) -> ()  [unwired: 7 in, 2 out]
                n131 = call "CTRE_Phoenix_MotorControl_Set.vi"("Output"=w323, "Control Mode"=w322, "PhoenixMotorControlDevRef"=w327) -> ()  [unwired: 7 in, 2 out]
                n132 = call "CTRE_Phoenix_MotorControl_Set.vi"("Output"=w323, "Control Mode"=w322, "PhoenixMotorControlDevRef"=w326) -> ()  [unwired: 7 in, 2 out]
              }
            }
          }
          frame condition #2 (active) {
          }
        }
        n133 = Less Or Equal To 0?(x=w282) -> (x <= 0?=w273:bool)
        n134 = Max & Min(x=w282, y=25.0) -> (min(x,y)=w278:dbl)  [unwired: 1 out]
        n135 = Or(x=w272, y=w273) -> (x .or. y?=w274:bool)
      }
      frame "Puke" {
        # "How much longer?\nUpdate motors every 25ms till time runs out OR\nsensor trips"
        n136 = Unbundle(w345) -> ("Start Time (ms)"=w348:u32, "Iterations"=w332:i32)
        n137 = Equal?(x=w332, y=0 ("value")) -> (x = y?=w330:bool)
        n138 = Subtract(x=w344, y=w348) -> (x-y=w351:u32)
        n139 = Multiply(x=w340, y=1000.0) -> (x*y=w350:dbl)
        n140 = case shown="True" w330 {
          tunnel: w329 -> [w352 w355]
          tunnel: [w352 w353] -> w328
          frame False {
          }
          frame True {
            n141 = call <vilib>:"WPI_AnalogTriggerGetOutput.vi"("AnalogTriggerDevRef"=w355) -> ("Trigger State"=→"WaitTrigger":bool, "AnalogTriggerDevRef"=w353:T5)  [unwired: 7 in, 2 out]
          }
        }
        n142 = Subtract(x=w350, y=w351) -> (x-y=w347:dbl)
        n143 = disable-structure shown="robot_simulation==off" {
          disable-tunnel: w342 -> [w363 w388 _]
          disable-tunnel: w341 -> [w358 w383 _]
          disable-tunnel: w336 -> [w362 w387 _]
          disable-tunnel: w333 -> [_ _ _]
          disable-tunnel: [w361 w386 _] -> w337
          disable-tunnel: w335 -> [w364 w389 _]
          disable-tunnel: w334 -> [w360 w385 _]
          disable-tunnel: w328 -> [w357 w382 _]
          frame condition #0 {
            n144 = local read "WaitTrigger"() -> (w359:bool)
            n145 = case shown="True" w359 {
              tunnel: w357 -> [w366 w369]
              tunnel: [w365 FALSE ("Trigger State")] -> w356
              frame False {
                n146 = call <vilib>:"WPI_AnalogTriggerGetOutput.vi"("AnalogTriggerDevRef"=w366) -> ("Trigger State"=w365:bool)  [unwired: 7 in, 3 out]
              }
              frame True {
                n147 = call <vilib>:"WPI_AnalogTriggerGetOutput.vi"("AnalogTriggerDevRef"=w369) -> ("Trigger State"=w367:bool)  [unwired: 7 in, 3 out]
                n148 = local write "WaitTrigger"(w367) -> ()
              }
            }
            n149 = case shown="False" w356 {
              tunnel: w363 -> [w375 w379]
              tunnel: w358 -> [w374 w378]
              tunnel: w362 -> [_ w376]
              tunnel: [TRUE FALSE] -> w361
              tunnel: w364 -> [w372 _]
              tunnel: w360 -> [_ _]
              frame True {
                w370 = T16 0 items=["PercentOutput"=0, "Position"=1, "Velocity"=2, "Current"=3, "Follower"=5, "MotionProfile"=6, "MotionMagic"=7, "MotionMagicArc"=8, "MotionProfileArc"=10, "Disabled"=15] ("Control Mode")
                w371 = 0.0 ("Output")
                n150 = call "CTRE_Phoenix_MotorControl_Set.vi"("Output"=w371, "Control Mode"=w370, "PhoenixMotorControlDevRef"=w372) -> ()  [unwired: 7 in, 2 out]
                n151 = call "CTRE_Phoenix_MotorControl_Set.vi"("Output"=w371, "Control Mode"=w370, "PhoenixMotorControlDevRef"=w375) -> ()  [unwired: 7 in, 2 out]
                n152 = call "CTRE_Phoenix_MotorControl_Set.vi"("Output"=w371, "Control Mode"=w370, "PhoenixMotorControlDevRef"=w374) -> ()  [unwired: 7 in, 2 out]
              }
              frame False {
                w377 = T16 0 items=["PercentOutput"=0, "Position"=1, "Velocity"=2, "Current"=3, "Follower"=5, "MotionProfile"=6, "MotionMagic"=7, "MotionMagicArc"=8, "MotionProfileArc"=10, "Disabled"=15] ("Control Mode")
                n153 = call "CTRE_Phoenix_MotorControl_Set.vi"("Output"=w376, "Control Mode"=w377, "PhoenixMotorControlDevRef"=w379) -> ()  [unwired: 7 in, 2 out]
                n154 = call "CTRE_Phoenix_MotorControl_Set.vi"("Output"=w376, "Control Mode"=w377, "PhoenixMotorControlDevRef"=w378) -> ()  [unwired: 7 in, 2 out]
              }
            }
          }
          frame condition #1 {
            n155 = local read "WaitTrigger"() -> (w384:bool)
            n156 = case shown="True" w384 {
              tunnel: w382 -> [w391 w394]
              tunnel: [w390 FALSE ("Trigger State")] -> w381
              frame False {
                n157 = call <vilib>:"WPI_AnalogTriggerGetOutput.vi"("AnalogTriggerDevRef"=w391) -> ("Trigger State"=w390:bool)  [unwired: 7 in, 3 out]
              }
              frame True {
                n158 = call <vilib>:"WPI_AnalogTriggerGetOutput.vi"("AnalogTriggerDevRef"=w394) -> ("Trigger State"=w392:bool)  [unwired: 7 in, 3 out]
                n159 = local write "WaitTrigger"(w392) -> ()
              }
            }
            n160 = case shown="False" w381 {
              tunnel: w388 -> [w400 w408]
              tunnel: w383 -> [w399 w407]
              tunnel: w387 -> [_ w402]
              tunnel: [TRUE FALSE] -> w386
              tunnel: w389 -> [w397 w406]
              tunnel: w385 -> [_ w404]
              frame True {
                w395 = T16 0 items=["PercentOutput"=0, "Position"=1, "Velocity"=2, "Current"=3, "Follower"=5, "MotionProfile"=6, "MotionMagic"=7, "MotionMagicArc"=8, "MotionProfileArc"=10, "Disabled"=15] ("Control Mode")
                w396 = 0.0 ("Output")
                n161 = call "CTRE_Phoenix_MotorControl_Set.vi"("Output"=w396, "Control Mode"=w395, "PhoenixMotorControlDevRef"=w397) -> ()  [unwired: 7 in, 2 out]
                n162 = call "CTRE_Phoenix_MotorControl_Set.vi"("Output"=w396, "Control Mode"=w395, "PhoenixMotorControlDevRef"=w400) -> ()  [unwired: 7 in, 2 out]
                n163 = call "CTRE_Phoenix_MotorControl_Set.vi"("Output"=w396, "Control Mode"=w395, "PhoenixMotorControlDevRef"=w399) -> ()  [unwired: 7 in, 2 out]
              }
              frame False {
                w405 = T16 0 items=["PercentOutput"=0, "Position"=1, "Velocity"=2, "Current"=3, "Follower"=5, "MotionProfile"=6, "MotionMagic"=7, "MotionMagicArc"=8, "MotionProfileArc"=10, "Disabled"=15] ("Control Mode")
                n164 = Negate(x=w404) -> (-x=w403:dbl)
                n165 = Negate(x=w402) -> (-x=w401:dbl)
                n166 = call "CTRE_Phoenix_MotorControl_Set.vi"("Output"=w401, "Control Mode"=w405, "PhoenixMotorControlDevRef"=w408) -> ()  [unwired: 7 in, 2 out]
                n167 = call "CTRE_Phoenix_MotorControl_Set.vi"("Output"=w401, "Control Mode"=w405, "PhoenixMotorControlDevRef"=w407) -> ()  [unwired: 7 in, 2 out]
                n168 = call "CTRE_Phoenix_MotorControl_Set.vi"("Output"=w403, "Control Mode"=w405, "PhoenixMotorControlDevRef"=w406) -> ()  [unwired: 7 in, 2 out]
              }
            }
          }
          frame condition #2 (active) {
          }
        }
        n169 = Less Or Equal To 0?(x=w347) -> (x <= 0?=w338:bool)
        n170 = Max & Min(x=w347, y=25.0) -> (min(x,y)=w343:dbl)  [unwired: 1 out]
        n171 = Or(x=w337, y=w338) -> (x .or. y?=w339:bool)
      }
    }
    n172 = call "cube Check for New Command.vi"("Current Command"=w79, "Wait time (ms)"=w67, "Finished?"=w68) -> ("Completion"=w80:T1, "Subsystem Name"=w81:string, "Current Command"=w82:T2, "Initial Trace String"=w83:string, "NextCommand"=w84:T15)  [unwired: 4 in]
    n173 = case shown="\"Successful\", \"Aborted\"" w80 {
      selector: w80 -> [_ w103]
      tunnel: w83 -> [_ w99]
      tunnel: w82 -> [_ w100]
      tunnel: w81 -> [_ w97]
      frame "Incomplete", Default {
        # "Continuing current command"
      }
      frame "Successful", "Aborted" {
        # "Report and setup for next command"
        n174 = Unbundle By Name(w100) -> ("Arm Setpoint"=w102:dbl, "Duration"=w96:dbl, "Conveyor Setpoint"=w95:dbl)
        n175 = Format Into String(format string="A %.1f, C %.1f, D %f", initial string=w99, w102, w95, w96) -> (resulting string=w98:string)  [unwired: 1 in, 1 out]
        "Current\nCmd" <- w98
        n176 = call <vilib>:"Trace Results.vi"("Status of previous command"=w103, "Description"=w98, "Subsystem"=w97) -> ()  [unwired: 9 in]
      }
    }
    n177 = disable-structure shown="Disabled" {
      frame Disabled {
        # "Publish"
        n178 = call-poly <vilib>:"NT Write Value.vi"() -> ()  [unwired: 11 in, 1 out]
      }
      frame Enabled {
      }
    }
  }
